vi "Memory Cell to rot3d.vi"(10 "Memory Cell":T1={"type"=enum."rotation", "x"=0.0, "y"=0.0, "z"=0.0, "w"=0.0}) -> (2 "Orient3d out":refnum<class "Orient3d.lvclass">)   [LabVIEW 2023]
uses:
  Type Definitions/Memory Cell.ctl
  Type Definitions/Memory Cell Type Enum.ctl
  Shared Components/Orient3d Class/Orient3d.lvclass
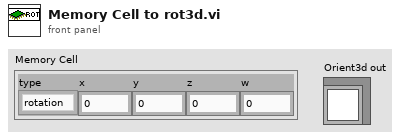
[diagram p1: front panel]
types:
  T1 = typedef "Memory Cell.ctl" = cluster{"type":T2, "x":dbl, "y":dbl, "z":dbl, "w":dbl}
  T2 = typedef "Memory Cell Type Enum.ctl" = enum16{"integer", "float", "vector", "rotation"}
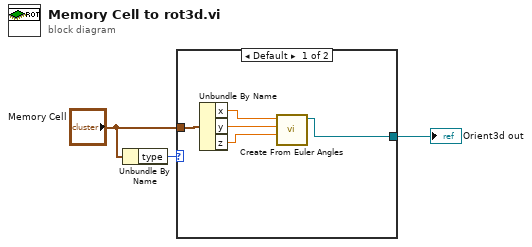
[diagram p0: block diagram]
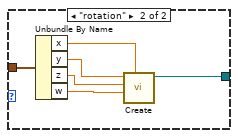
[diagram p2: hidden frame]
diagram:
  n1 = Unbundle By Name("Memory Cell") -> ("type"=w1:T2)
  n2 = case shown="Default" w1 {
    tunnel: "Memory Cell" -> [w8 w14]
    tunnel: [w4 w9] -> w3
    frame Default {
      n3 = Unbundle By Name(w8) -> ("x"=w7:dbl, "y"=w6:dbl, "z"=w5:dbl)
      n4 = call "Create From Euler Angles.vi"("phi/roll"=w5, "theta/pitch"=w6, "psi/yaw"=w7) -> ("Orient3d out"=w4:refnum<class "Orient3d.lvclass">)  [unwired: 7 in, 1 out]
    }
    frame "rotation" {
      n5 = Unbundle By Name(w14) -> ("x"=w10:dbl, "y"=w11:dbl, "z"=w12:dbl, "w"=w13:dbl)
      n6 = call "Create.vi"("x"=w10, "w"=w13, "z"=w12, "y"=w11) -> ("Orient3d out"=w9:refnum<class "Orient3d.lvclass">)  [unwired: 6 in, 1 out]
    }
  }
  "Orient3d out" <- w3
